vi "Set Baud.vi"(8 "error in (no error)":errorcluster, 9 "New Baud":u32=38400, 10 "Old Baud":u32=115200, 11 "COM Port":refnum<visa-resource-name>="COM4") -> (0 "error out":errorcluster, 3 "Result":bool)   [LabVIEW 2018]
panel:
  out "Size Array":u16
  out "Data Array":u8[](array[numeric]) format="%x"
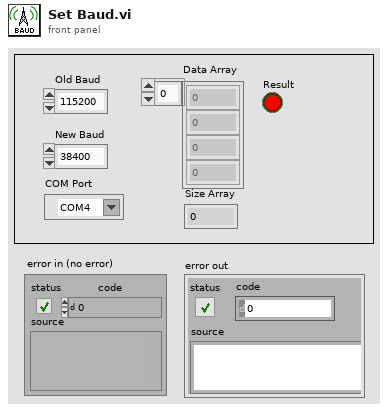
[diagram p1: front panel]
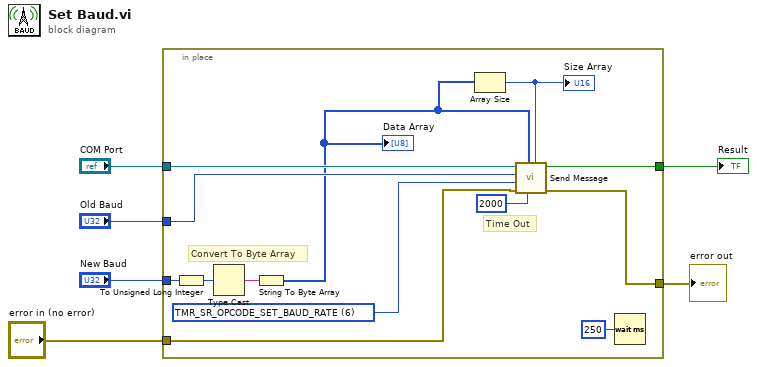
[diagram p0: block diagram]
diagram:
  n1 = in-place {
    in-place-border: "New Baud" -> [w19]
    in-place-border: "COM Port" -> [w17]
    in-place-border: "Old Baud" -> [w16]
    in-place-border: [w13] -> w3
    in-place-border: [w12] -> w2
    in-place-border: "error in (no error)" -> [w8]
    w11 = u16 6 items=["TMR_SR_OPCODE_VERSION"=3, "TMR_SR_OPCODE_SET_BAUD_RATE"=6, "TMR_SR_OPCODE_READ_TAG_ID_SINGLE"=33, "TMR_SR_OPCODE_READ_TAG_ID_MULTIPLE"=34, "TMR_SR_OPCODE_WRITE_TAG_ID"=35, "TMR_SR_OPCODE_WRITE_TAG_DATA"=36, "TMR_SR_OPCODE_KILL_TAG"=38, "TMR_SR_OPCODE_READ_TAG_DATA"=40, "TMR_SR_OPCODE_CLEAR_TAG_ID_BUFFER"=42, "TMR_SR_OPCODE_MULTI_PROTOCOL_TAG_OP"=47, "TMR_SR_OPCODE_GET_READ_TX_POWER"=98, "TMR_SR_OPCODE_GET_WRITE_TX_POWER"=100, "TMR_SR_OPCODE_GET_POWER_MODE"=104, "TMR_SR_OPCODE_GET_READER_OPTIONAL_PARAMS"=106, "TMR_SR_OPCODE_GET_PROTOCOL_PARAM"=107, "TMR_SR_OPCODE_SET_ANTENNA_PORT"=145, "TMR_SR_OPCODE_SET_TAG_PROTOCOL"=147, "TMR_SR_OPCODE_SET_READ_TX_POWER"=146, "TMR_SR_OPCODE_SET_WRITE_TX_POWER"=148, "TMR_SR_OPCODE_SET_REGION"=151, "TMR_SR_OPCODE_SET_READER_OPTIONAL_PARAMS"=154, "TMR_SR_OPCODE_SET_PROTOCOL_PARAM"=155] ("Opcode Constant")
    # "Convert To Byte Array"
    # "Time Out"
    n2 = To Unsigned Long Integer(number=w19) -> (unsigned 32bit integer=w18:u32)
    n3 = Type Cast(x=w18) -> (*(type *) &x=w10:string)  [unwired: 1 in]
    n4 = String To Byte Array(string=w10) -> (unsigned byte array=w9:u8[])
    "Data Array" <- w9
    n5 = Array Size(array=w9) -> (size(s)=w15:i32)
    "Size Array" <- w15
    n6 = call "Send Message.vi"("Size"=w15, "timeOut (ms)"=u32 2000, "Data"=w9, "error in (no error)"=w8, "Opcode"=w11, "Baud Rate"=w16, "COM Port"=w17) -> ("error out"=w12:errorcluster, "Result"=w13:bool)  [unwired: 1 in, 2 out]
    n7 = Wait (ms)(milliseconds to wait=u32 250) -> ()  [unwired: 1 out]
  }
  "Result" <- w3
  "error out" <- w2
